vi "eFGV - AO Data RT.vi"(6 "States":T1, 8 "Error In":errorcluster, 11 "AO Data":dbl[](array[numeric])) -> (0 "Error Out":errorcluster, 2 "Event AO Data":refnum<user-event>, 3 "AO Data Out":dbl[](array[numeric]))   [LabVIEW 2020]
uses:
  Control/State - eFGV.ctl
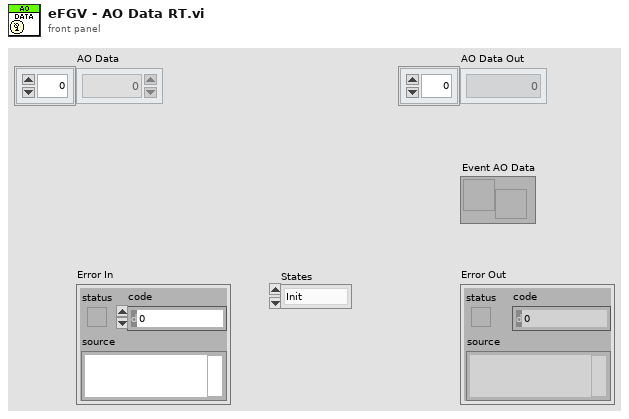
[diagram p1: front panel]
types:
  T1 = typedef "State - eFGV.ctl" = enum16{"Init", "Read", "Write", "Exit"}
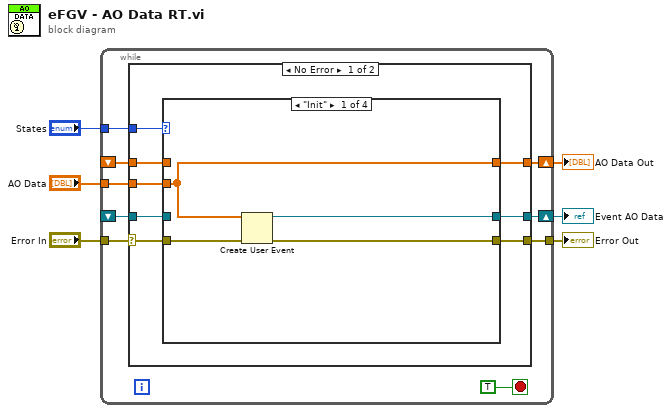
[diagram p0: block diagram]
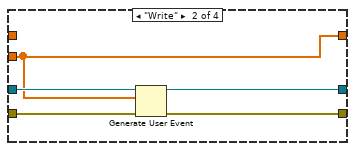
[diagram p2: hidden frame]
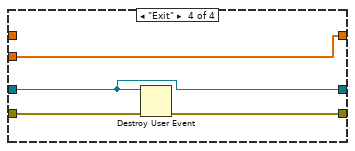
[diagram p4: hidden frame]
diagram:
  n1 = while {
    tunnel: "Error In" -> [w15]
    tunnel: [w14] -> w5
    tunnel: "States" -> [w12]
    tunnel: "AO Data" -> [w11]
    shift-right: [w10] -> w2
    shift-left: _ -> [w9]
    shift-right: [w8] -> w1
    shift-left: _ -> [w7]
    stop <- TRUE stop-if-true
    n2 = case shown="No Error" w15 {
      selector: w15 -> [w23 w42]
      tunnel: [w22 w42] -> w14
      tunnel: w12 -> [w21 _]
      tunnel: w11 -> [w20 w40]
      tunnel: [w19 w41] -> w10
      tunnel: w9 -> [w18 w41]
      tunnel: [w17 w40] -> w8
      tunnel: w7 -> [w16 _]
      frame No Error {
        n3 = case shown="\"Init\"" w21 {
          tunnel: w23 -> [w27 w32 w35 w39]
          tunnel: [w26 w31 w35 w38] -> w22
          tunnel: w20 -> [w24 w28 _ w36]
          tunnel: [w25 w29 w34 w37] -> w19
          tunnel: w18 -> [_ w30 w34 w37]
          tunnel: [w24 w28 w33 w36] -> w17
          tunnel: w16 -> [_ _ w33 _]
          frame "Init" {
            n4 = Create User Event(user event datatype=w24, error in=w27) -> (user event=w25:refnum<user-event>, error out=w26:errorcluster)
          }
          frame "Write" {
            n5 = Generate User Event(user event=w30, event data cluster=w28, error in=w32) -> (user event out=w29:refnum<user-event>, error out=w31:errorcluster)  [unwired: 1 in]
          }
          frame "Read" {
          }
          frame "Exit" {
            n6 = Destroy User Event(user event=w37, error in=w39) -> (error out=w38:errorcluster)
          }
        }
      }
      frame Error {
      }
    }
  }
  "Error Out" <- w5
  "Event AO Data" <- w2
  "AO Data Out" <- w1
